vi "Lvi Bridge Sensor Channel Settings.vi"(0 "TaskRef":i32, 1 "TransducerCapacity":dbl, 2 "GageResistance":dbl, 3 "UnstrainedVoltage":dbl, 5 "Channel":u32, 7 "BridgeExcitationSource":i32, 9 "ExcitationVoltage":dbl, 11 "error in (no error)":errorcluster, 12 "RatedOutput":dbl, 13 "WireResistance":dbl, 14 "ShuntCorrection":dbl) -> (4 "TaskRef out":i32, 6 "function return":i32, 15 "error out":errorcluster)   [LabVIEW 2022 SP3, in "DtLvLink.lvlib"]
doc: "Calls directly into the entry points of the DLL of the Data Acq SDK to return TEDS information about a bridge-based sensor."
uses:
  DtLvLink.lvlib
  <userlib>/LV-Link3/DtLvLink_64.dll
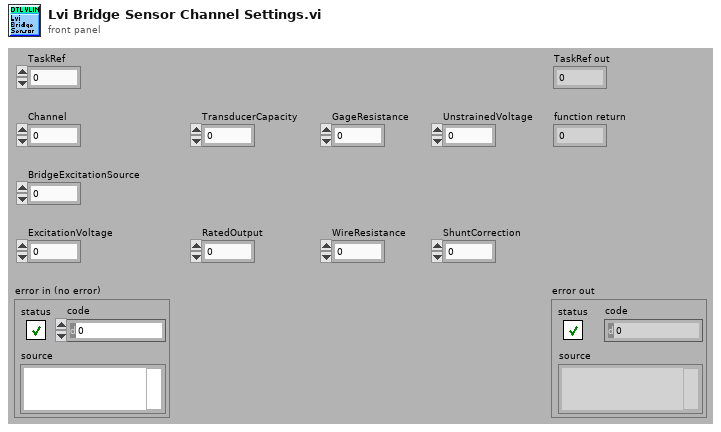
[diagram p1: front panel]
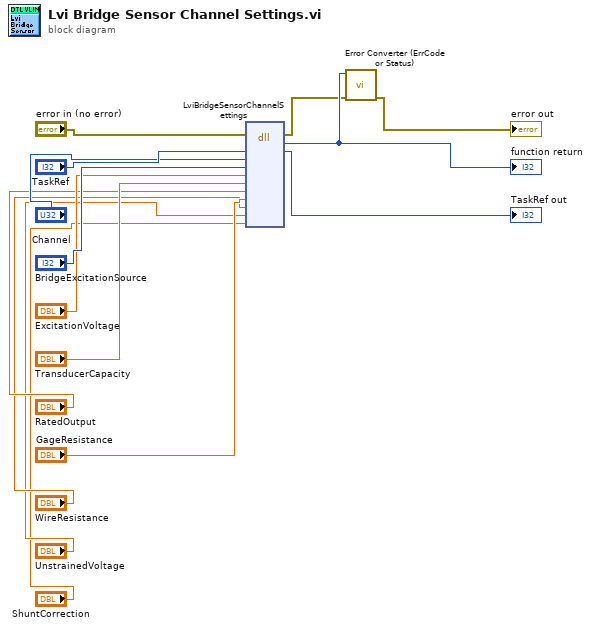
[diagram p0: block diagram]
diagram:
  n1 = dll-call lib="C:/Program Files/National Instruments/LabVIEW 2022/user.lib/LV-Link3/DtLvLink_64.*" fn="LviBridgeSensorChannelSettings"(error in="error in (no error)", "TaskRef"="TaskRef", "Channel"="Channel", "BridgeExcitationSource"="BridgeExcitationSource", "ExcitationVoltage"="ExcitationVoltage", "TransducerCapacity"="TransducerCapacity", "RatedOutput"="RatedOutput", "GageResistance"="GageResistance", "WireResistance"="WireResistance", "UnstrainedVoltage"="UnstrainedVoltage", "ShuntCorrection"="ShuntCorrection") -> (error out=w2:errorcluster, "return type"=w15:i32, "TaskRef"=→"TaskRef out":i32)  [unwired: 11 in, 1 out]
  "function return" <- w15
  n2 = call "Error Converter (ErrCode or Status).vi"("error in (no error)"=w2, "error code"=w15) -> ("error out"=→"error out":errorcluster)  [unwired: 9 in]
